vi "Load Class by Name.vi"(5 "Class Type":refnum<class>, 8 "error in (no error)":errorcluster, 11 "Base Class Name":string) -> (0 "error out":errorcluster, 1 "Load and Type Success?":bool, 2 "Class load Success?":bool, 3 "Loaded Class":refnum<class>)   [LabVIEW 2019, in "ClassLoader.lvlib"]
doc: "Load a named class from the cache by getting the class path. If the cache does not contain the class name it is refreshed.\nAfter class load it is casted to the given 'Class Type' using Preserve Run-Time Class."
uses:
  ClassLoader.lvlib
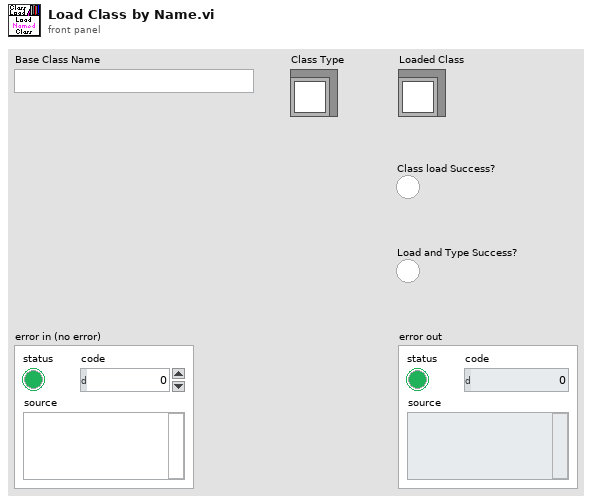
[diagram p1: front panel]
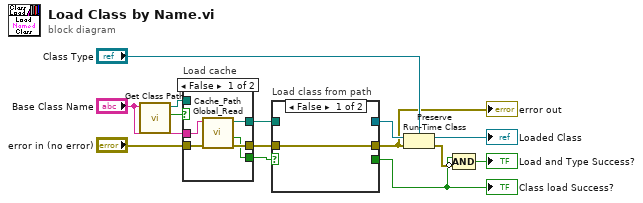
[diagram p0: block diagram]
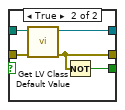
[diagram p3: hidden frame]
diagram:
  n1 = call "Get Class Path.vi"("Base Class Name"="Base Class Name") -> ("Success?"=w2:bool, "Path"=w1:path)  [unwired: 9 in]
  n2 = case "Load cache" shown="False" w2 {
    selector: w2 -> [_ w20]
    tunnel: "error in (no error)" -> [w19 w21]
    tunnel: [w18 w21] -> w7
    tunnel: [w17 w20] -> w6
    tunnel: [w16 w22] -> w5
    tunnel: "Base Class Name" -> [w15 _]
    tunnel: w1 -> [_ w22]
    frame False {
      n3 = call "Cache_Path Global_Read.vi"("error in (no error)"=w19, "Class Name"=w15) -> ("error out"=w18:errorcluster, "Success?"=w17:bool, "Class Path"=w16:path)  [unwired: 7 in]
    }
    frame True {
    }
  }
  n4 = case "Load class from path" shown="False" w6 {
    tunnel: w5 -> [_ w28]
    tunnel: [_ w27] -> w14
    tunnel: w7 -> [w23 w26]
    tunnel: [w23 w25] -> w11
    tunnel: [_ w24] -> w4
    frame False {
    }
    frame True {
      n5 = call <vilib>:"Get LV Class Default Value.vi"("error in (no error)"=w26, "class path"=w28) -> ("error out"=w25:errorcluster, "object"=w27:refnum<class>)  [unwired: 8 in]
      n6 = Not(x=w25) -> (.not. x?=w24:bool)
    }
  }
  "error out" <- w11
  "Class load Success?" <- w4
  n7 = Preserve Run-Time Class(object in=w14, error in=w11, 2:"Class Type") -> (object out=→"Loaded Class":refnum<class>, error out=w10:errorcluster)
  n8 = Compound Arithmetic op=AND(w4, invert w10) -> (→"Load and Type Success?":bool)
